vi "CreateFile.vi"(11 "Date/Time":string) -> (0 "error out":errorcluster, 2 "Date/Time String":string, 3 "Refnum Out":refnum<file>)   [LabVIEW 2017]
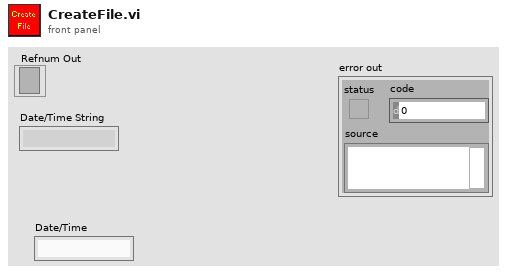
[diagram p1: front panel]
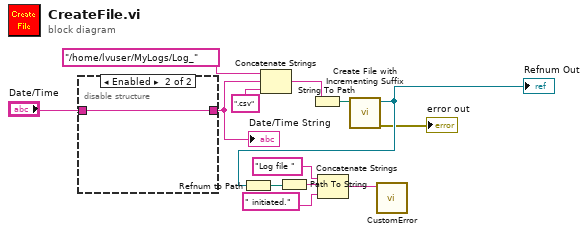
[diagram p0: block diagram]
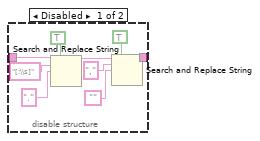
[diagram p2: hidden frame]
diagram:
  n1 = disable-structure shown="Enabled" {
    disable-tunnel: [w22 w23] -> w7
    disable-tunnel: "Date/Time" -> [w14 w23]
    frame Disabled {
      n2 = Search and Replace String(replace all?=TRUE ("replace all? (F)"), input string=w14, search string="[:\\s]", replace string="." ("replace string (\"\")")) -> (result string=w18:string)  [unwired: 4 in, 3 out]
      n3 = Search and Replace String(replace all?=TRUE ("replace all? (F)"), input string=w18, search string=",", replace string="") -> (result string=w22:string)  [unwired: 4 in, 3 out]
    }
    frame Enabled {
    }
  }
  "Date/Time String" <- w7
  n4 = Concatenate Strings("/home/lvuser/MyLogs/Log_" ("string"), w7, ".csv" ("string")) -> (w5:string)
  n5 = String To Path(string=w5) -> (path=w6:path)
  n6 = call <vilib>:"Create File with Incrementing Suffix.vi"("file path"=w6) -> ("error out"=→"error out":errorcluster, "refnum out"=w10:refnum<file>)  [unwired: 8 in, 1 out]
  "Refnum Out" <- w10
  n7 = Refnum to Path(1:w10) -> (0:w9:path)
  n8 = Path To String(path=w9) -> (string=w11:string)
  n9 = Concatenate Strings("Log file " ("Source"), w11, " initiated." ("string")) -> (w13:string)
  n10 = call "CustomError.vi"("String"=w13) -> ()  [unwired: 10 in, 1 out]
